vi "Pre-Scan Check.vi"(8 "error in (no error)":errorcluster, 10 "Current scan #":i32, 11 "Scan Driver in":refnum<class "Scan Driver.lvclass">) -> (0 "error out":errorcluster, 3 "Scan Driver out":refnum<class "Scan Driver.lvclass">)   [LabVIEW 2009, in "Scan Driver.lvclass"]
doc: "Call \"Scan Setup\" on all Instruments contained in this Scan Driver instance. This will configure the Instruments according to their member fields. Move the Scanner to the First Step."
uses:
  Scan Driver.lvclass
  <vilib>/Utility/error.llb/DialogType.ctl
  Scan Driver.lvclass/Scan Driver.ctl
  Scanners/Scanner/Scanner.lvclass
  Readers/Reader/Reader.lvclass
panel:
  out "done":bool=TRUE
  out "current":string
  out "Busy Bar":bool[](array[boolean])
  # "Checking Instrument Status versus Desired Settings and Setting as Required"
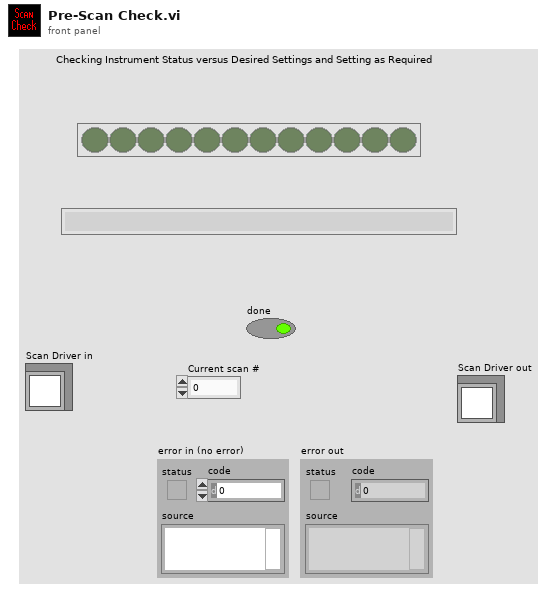
[diagram p1: front panel]
types:
  T1 = typedef "DialogType.ctl" = u16
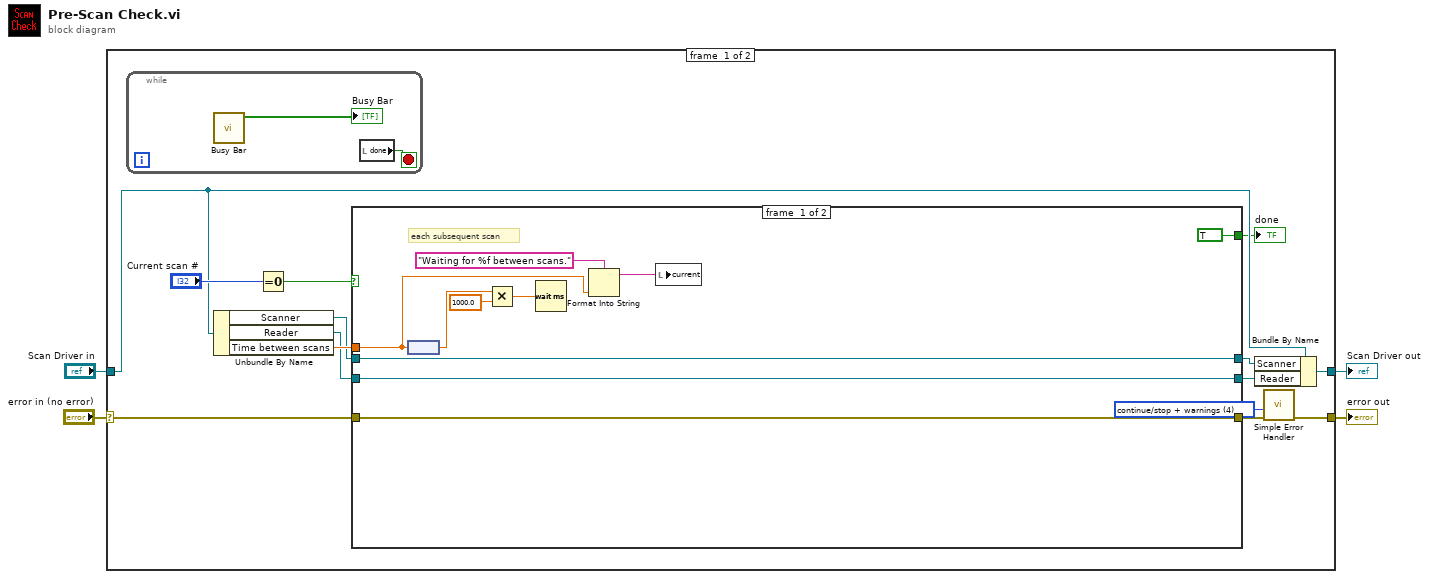
[diagram p0: block diagram]
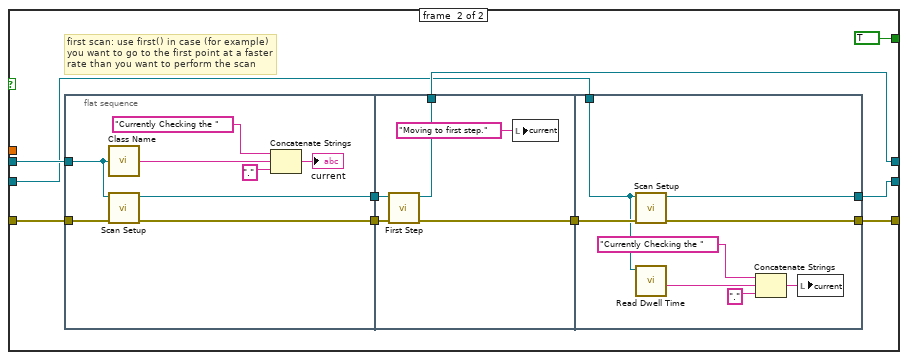
[diagram p2: hidden frame]
diagram:
  n1 = case shown="No Error" "error in (no error)" {
    selector: "error in (no error)" -> [w11 w63]
    tunnel: [w6 w63] -> w3
    tunnel: [w8 w62] -> w1
    tunnel: "Scan Driver in" -> [w10 w62]
    frame #0 {
      w5 = T1 4 items=["no dialog", "OK message", "continue or stop message", "OK message + warnings", "continue/stop + warnings"] ("type of dialog (OK msg:1)")
      n2 = while {
        stop <- w61 stop-if-true
        n3 = call "Busy Bar.vi"() -> ("Busy Bar"=→"Busy Bar":bool[])  [unwired: 2 in, 9 out]
        n4 = local read "done"() -> (w61:bool)
      }
      n5 = Unbundle By Name(w10) -> ("Scanner"=w15:refnum<class "Scanner.lvclass">, "Reader"=w14:refnum<class "Reader.lvclass">, "Time between scans"=w16:dbl[unit])
      n6 = Equal To 0?(x="Current scan #") -> (x = 0?=w18:bool)
      n7 = case shown="True" w18 {
        tunnel: w16 -> [w21 _]
        tunnel: w15 -> [w25 w38]
        tunnel: w11 -> [w24 w37]
        tunnel: [w25 w34] -> w12
        tunnel: [w24 w30] -> w7
        tunnel: w14 -> [w23 w32]
        tunnel: [w23 w31] -> w13
        tunnel: [TRUE TRUE] -> w9
        frame #0 {
          # "each subsequent scan"
          n8 = node(w21) -> (w28:dbl)
          n9 = Multiply(x=w28, y=1000.0) -> (x*y=w26:dbl)
          n10 = Wait (ms)(milliseconds to wait=w26) -> ()  [unwired: 1 out]
          n11 = Format Into String(format string="Waiting for %f between scans.", w21) -> (resulting string=w20:string)  [unwired: 2 in, 1 out]
          n12 = local write "current"(w20) -> ()
        }
        frame #1 {
          # "first scan: use first() in case (for example)\nyou want to go to the first point at a faster\nrate than you want to perform the scan"
          n13 = flat-sequence {
            tunnel: w38 -> [w45]
            tunnel: w37 -> [w46]
            tunnel: [w40] -> w36
            tunnel: [w39] -> w35
            tunnel: w36 -> [w50]
            tunnel: w35 -> [w49]
            tunnel: [w48] -> w34
            tunnel: [w47] -> w33
            tunnel: w33 -> [w56]
            tunnel: w32 -> [w52]
            tunnel: [w55] -> w31
            tunnel: [w54] -> w30
            frame #0 {
              n14 = call "Class Name.vi"("LabVIEW Object"=w45) -> ("Classname"=w41:string)
              n15 = call-dynamic "Scan Setup.vi"("error in (no error)"=w46, "Scanner in"=w45) -> ("error out"=w39:errorcluster, "Scanner out"=w40:refnum<class "Scanner.lvclass">)  [unwired: 8 out]
              n16 = Concatenate Strings("Currently Checking the ", w41, ".") -> (→"current":string)
            }
            frame #1 {
              n17 = call-dynamic "First Step.vi"("error in (no error)"=w49, "Scanner.lvclass in"=w50) -> ("error out"=w47:errorcluster, "Scanner.lvclass out"=w48:refnum<class "Scanner.lvclass">)  [unwired: 8 out]
              n18 = local write "current"("Moving to first step." ("current")) -> ()
            }
            frame #2 {
              n19 = call-dynamic "Scan Setup.vi"("error in (no error)"=w56, "Reader in"=w52) -> ("error out"=w54:errorcluster, "Reader out"=w55:refnum<class "Reader.lvclass">)  [unwired: 8 out]
              n20 = call-dynamic "Read Dwell Time.vi"("Reader.lvclass in"=w52) -> ("Most Specific Classname"=w53:string)  [unwired: 1 in, 9 out]
              n21 = Concatenate Strings("Currently Checking the ", w53, ".") -> (w57:string)
              n22 = local write "current"(w57) -> ()
            }
          }
        }
      }
      "done" <- w9
      n23 = Bundle By Name(cluster=w10, "Scanner"=w12, "Reader"=w13) -> (w8:refnum<class "Scan Driver.lvclass">)
      n24 = call <vilib>:"Simple Error Handler.vi"("type of dialog (OK msg:1)"=w5, "error in (no error)"=w7) -> ("error out"=w6:errorcluster)  [unwired: 7 out]
    }
    frame #1 {
    }
  }
  "error out" <- w3
  "Scan Driver out" <- w1
